vi "popup_(SubVI).vi"(1 "X":i32) -> (0 "Boolean":bool)   [LabVIEW 2020]
panel:
  in  "?":bool
  in  "?":bool
  out "?":string
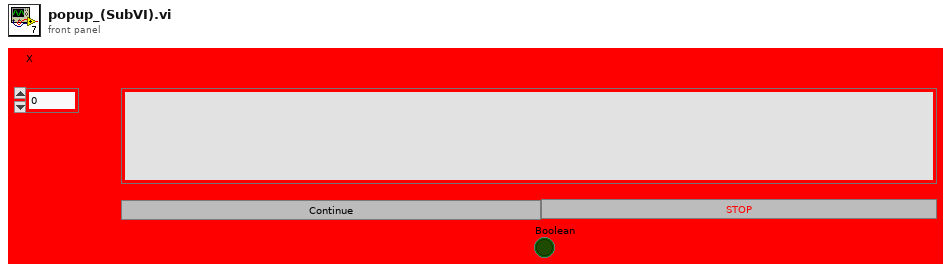
[diagram p1: front panel]
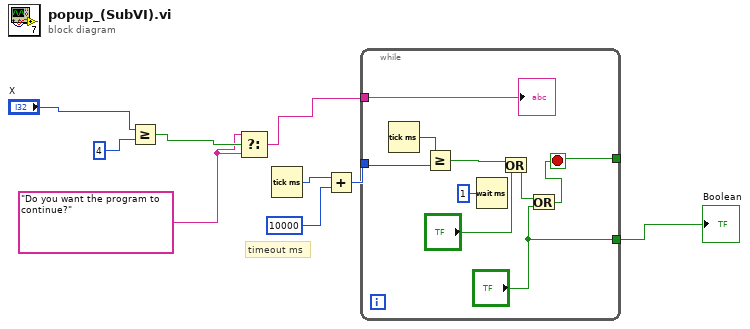
[diagram p0: block diagram]
diagram:
  w1 = "Do you want the program to continue?" ("f")
  # "timeout ms"
  n1 = Greater Or Equal?(x="X", y=4) -> (x >= y?=w5:bool)
  n2 = Select(t=w1, s=w5, f=w1) -> (s? t:f=w6:string)
  n3 = Tick Count (ms)() -> (millisecond timer value=w7:u32)
  n4 = Add(x=w7, y=u32 10000) -> (x+y=w8:u32)
  n5 = while {
    tunnel: w8 -> [w17]
    tunnel: [w11] -> _
    tunnel: w6 -> [w13]
    tunnel: ["?"] -> w2
    stop <- w11 stop-if-true
    n6 = Tick Count (ms)() -> (millisecond timer value=w16:u32)
    n7 = Greater Or Equal?(x=w16, y=w17) -> (x >= y?=w15:bool)
    n8 = Wait (ms)(milliseconds to wait=u32 1 ("millisecond timer value")) -> ()  [unwired: 1 out]
    n9 = Or(x=w15, y="?") -> (x .or. y?=w12:bool)
    n10 = Or(x=w12, y="?") -> (x .or. y?=w11:bool)
    "?" <- w13
  }
  "Boolean" <- w2
